vi "runtest calculate repeat run.vi"(1 "SeqCount":u32, 2 "Repeat N":u32) -> (0 "RUN?":bool)   [LabVIEW 2011]
panel:
  # "We should execute this step:\n\n0)  First sequence exection only;\n1)  Every sequence execution;\n2)  Every other sequence execution (0, 2, 4, ...)\n3)  Every third sequence execution (0, 3, 6, ...)\n4)  Every fourth sequence execution (0, 4, 8,...)\n\nand so on..."
  # "How many times has\nsequence been executed\nthis session?"
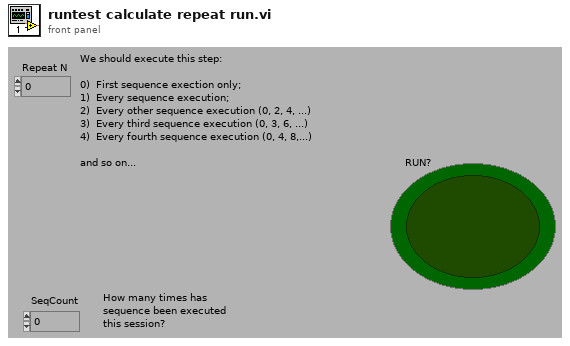
[diagram p1: front panel]
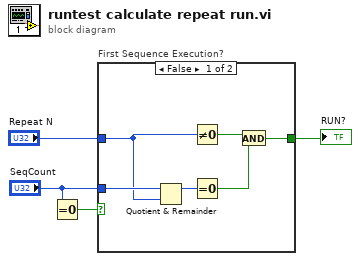
[diagram p0: block diagram]
diagram:
  n1 = Equal To 0?(x="SeqCount") -> (x = 0?=w1:bool)
  n2 = case "First Sequence Execution?" shown="False" w1 {
    selector: w1 -> [_ w11]
    tunnel: "Repeat N" -> [w5 _]
    tunnel: [w7 w11] -> w3
    tunnel: "SeqCount" -> [w6 _]
    frame False {
      n3 = Quotient & Remainder(x=w6, y=w5) -> (x-y*floor(x/y)=w10:u32)  [unwired: 1 out]
      n4 = Not Equal To 0?(x=w5) -> (x != 0?=w9:bool)
      n5 = Equal To 0?(x=w10) -> (x = 0?=w8:bool)
      n6 = And(x=w9, y=w8) -> (x .and. y?=w7:bool)
    }
    frame True {
    }
  }
  "RUN?" <- w3
